vi "OnImageFrameAvailable Event Callback - 16-bit.vi"(4 "User Parameter":T1, 5 "Event Data":T2, 6 "Control Ref":refnum<k24>, 7 "Event Common Data":T3) -> ()   [LabVIEW 2015]
uses:
  C:/code/ScientificCameraInterfaces/Installer/Scientific Camera Interfaces/LabVIEW/32_bit/Library_X86/Thorlabs.TSI.TLCameraInterfaces.dll
  code/ScientificCameraInterfaces/Installer/Scientific Camera Interfaces/LabVIEW/32_bit/Library_X86/Thorlabs.TSI.TLCameraInterfaces.dll
  C:/code/ScientificCameraInterfaces/Installer/Scientific Camera Interfaces/LabVIEW/32_bit/Library_X86/Thorlabs.TSI.ImageData.dll
  code/ScientificCameraInterfaces/Installer/Scientific Camera Interfaces/LabVIEW/32_bit/Library_X86/Thorlabs.TSI.ImageData.dll
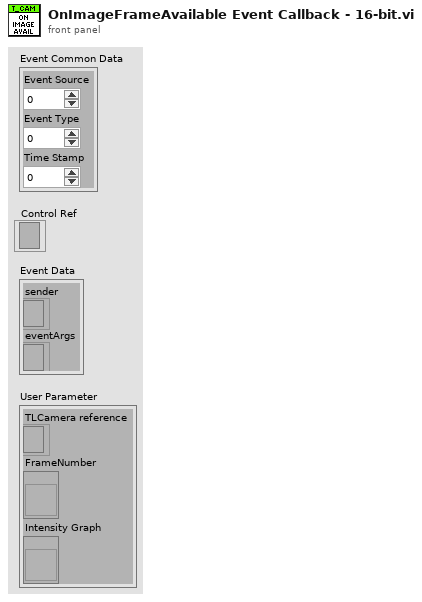
[diagram p1: front panel]
types:
  T1 = cluster{"TLCamera reference":refnum<k24>, "FrameNumber":refnum<vi>, "Intensity Graph":refnum<vi>}
  T2 = cluster{"sender":refnum<k24>, "eventArgs":refnum<k24>}
  T3 = cluster{"Event Source":i32, "Event Type":u32, "Time Stamp":u32}
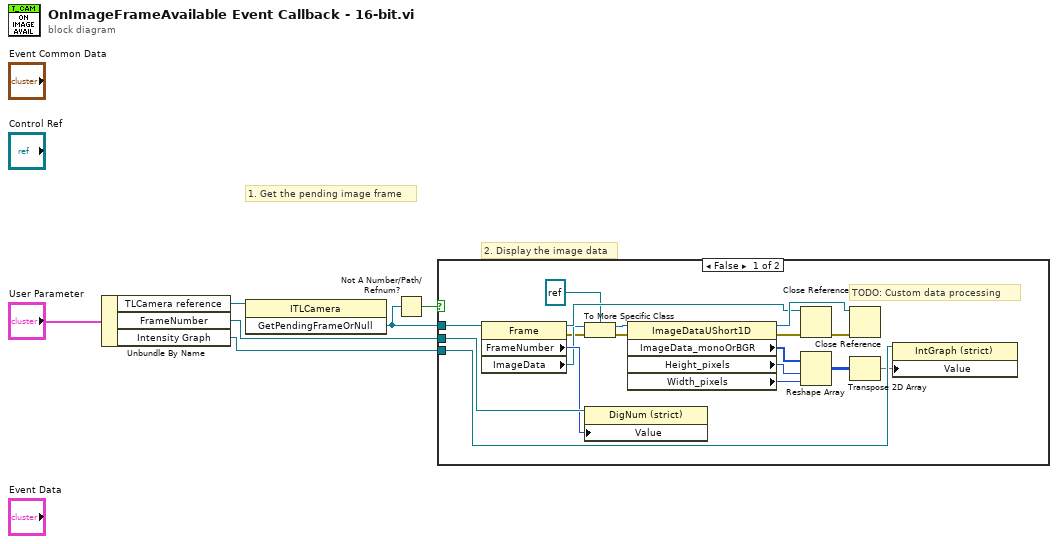
[diagram p0: block diagram]
diagram:
  # "2. Display the image data"
  # "1. Get the pending image frame"
  n1 = Unbundle By Name("User Parameter") -> ("TLCamera reference"=w3:refnum<k24>, "FrameNumber"=w2:refnum<vi>, "Intensity Graph"=w1:refnum<vi>)
  n2 = invoke class="ITLCamera" method="GetPendingFrameOrNull"(reference=w3) -> ("GetPendingFrameOrNull"=w5:refnum<k24>)  [unwired: 2 in, 2 out]
  n3 = Not A Number/Path/Refnum?(number/path/refnum=w5) -> (NaN/Path/Refnum?=w6:bool)
  n4 = case shown="False" w6 {
    tunnel: w5 -> [w24 _]
    tunnel: w2 -> [w23 _]
    tunnel: w1 -> [w21 _]
    frame False {
      # "TODO: Custom data processing"
      n5 = property class="Frame"(reference=w24) -> (reference out=w16:refnum<k24>, error out=w11:errorcluster, "FrameNumber"=w22:u32, "ImageData"=w12:refnum<k24>)  [unwired: 1 in]
      n6 = To More Specific Class(target class=refnum<k24> refnum, reference=w12, error in=w11) -> (specific class reference=w9:refnum<k24>, error out=w8:errorcluster)
      n7 = property class="DigNum (strict)"(reference=w23, "Value"=w22) -> ()  [unwired: 1 in, 2 out]
      n8 = property class="ImageDataUShort1D"(reference=w9, error in=w8) -> (reference out=w17:refnum<k24>, error out=w19:errorcluster, "ImageData_monoOrBGR"=w20:u16[], "Height_pixels"=w15:i32, "Width_pixels"=w14:i32)
      n9 = Close Reference(reference=w16, error in (no error)=w19) -> (error out=w18:errorcluster)
      n10 = Reshape Array(w20, w15, w14) -> (w7:u16[][])
      n11 = Close Reference(reference=w17, error in (no error)=w18) -> ()  [unwired: 1 out]
      n12 = Transpose 2D Array(2D array=w7) -> (transposed array=w13:u16[][])
      n13 = property class="IntGraph (strict)"(reference=w21, "Value"=w13) -> ()  [unwired: 1 in, 2 out]
    }
    frame True {
    }
  }
